vi "Shoot Joystick.vi"(6 "Auto Calculate Speed":bool, 8 "Trench Speed":bool, 9 "Init LIne Speed":bool, 10 "Target Zone Speed":bool, 11 "Raw Throttle":dbl) -> (3 "Shoot Teleop Command":T1)   [LabVIEW 2019]
uses:
  Shooter Mode Type Def.ctl
  Shooter Command Type Def.ctl
  Shooter Preset speeds Type Def.ctl
panel:
  # "AUTO CALCULATE DOES NOT DO\nANYTHING RIGHT NOW"
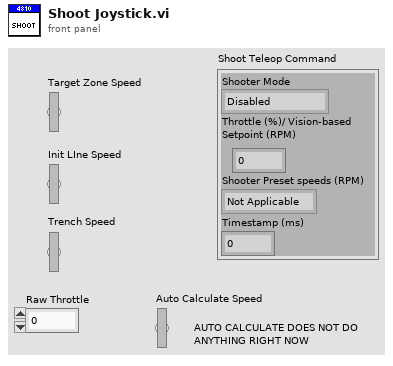
[diagram p1: front panel]
types:
  T1 = typedef "Shooter Command Type Def.ctl" = cluster{"Shooter Mode":T2, "Throttle (%)/ Vision-based\nSetpoint (RPM)":dbl, "Shooter Preset speeds (RPM)":T3, "Timestamp (ms)":dbl}
  T2 = typedef "Shooter Mode Type Def.ctl" = enum16{"Disabled", "Raw Throttle", "Preset Velocity Control", "Vision-based Velocity Control"}
  T3 = typedef "Shooter Preset speeds Type Def.ctl" = enum16{"Not Applicable", "Target Zone", "Initiation Line", "Close end of Trench Run", "Control Panel"}
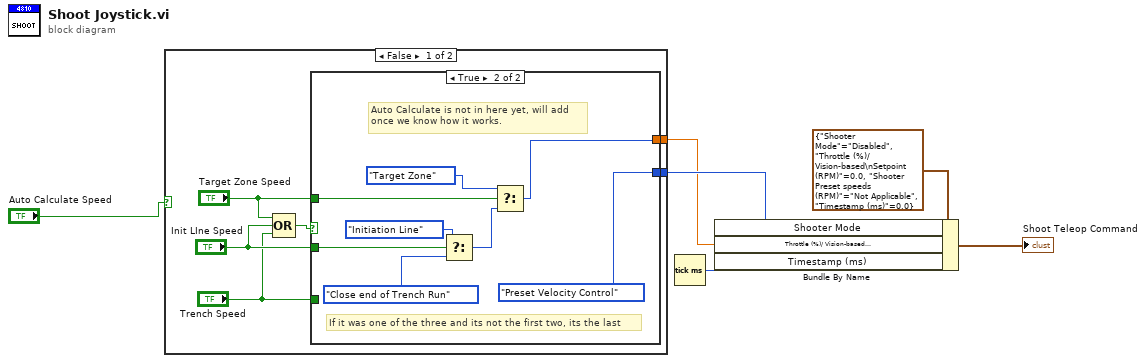
[diagram p0: block diagram]
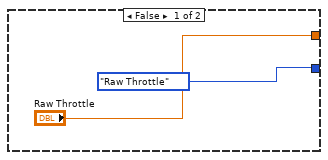
[diagram p2: hidden frame]
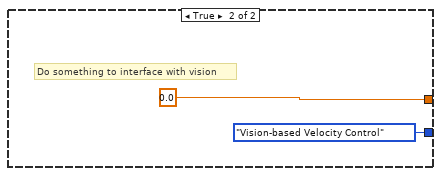
[diagram p3: hidden frame]
diagram:
  n1 = case shown="False" "Auto Calculate Speed" {
    tunnel: [w12 Shooter_Mode_Type_Def."Vision-based Velocity Control" ("Shooter Mode")] -> w3
    tunnel: [w7 0.0 ("Raw Throttle")] -> w2
    frame False {
      n2 = Compound Arithmetic op=OR("Target Zone Speed", "Init LIne Speed", "Trench Speed") -> (w11:bool)
      n3 = case shown="True" w11 {
        tunnel: "Trench Speed" -> [_ _]
        tunnel: "Init LIne Speed" -> [_ w22]
        tunnel: "Target Zone Speed" -> [_ w21]
        tunnel: [Shooter_Mode_Type_Def."Raw Throttle" ("Shooter Mode") Shooter_Mode_Type_Def."Preset Velocity Control" ("Shooter Mode")] -> w12
        tunnel: ["Raw Throttle" w19] -> w7
        frame False {
        }
        frame True {
          # "If it was one of the three and its not the first two, its the last"
          # "Auto Calculate is not in here yet, will add\nonce we know how it works."
          n4 = Select(t=Shooter_Preset_speeds_Type_Def."Initiation Line" ("Shooter Preset speeds (RPM)"), s=w22, f=Shooter_Preset_speeds_Type_Def."Close end of Trench Run" ("Shooter Preset speeds (RPM)")) -> (s? t:f=w20:T3)
          n5 = Select(t=Shooter_Preset_speeds_Type_Def."Target Zone" ("Shooter Preset speeds (RPM)"), s=w21, f=w20) -> (s? t:f=w19:T3)
        }
      }
    }
    frame True {
      # "Do something to interface with vision"
    }
  }
  n6 = Tick Count (ms)() -> (millisecond timer value=w4:u32)
  n7 = Bundle By Name(cluster=T1 {"Shooter Mode"=enum."Disabled", "Throttle (%)/ Vision-based\nSetpoint (RPM)"=0.0, "Shooter Preset speeds (RPM)"=enum."Not Applicable", "Timestamp (ms)"=0.0} ("Teleop Shooter Command"), "Shooter Mode"=w3, "Throttle (%)/ Vision-based\nSetpoint (RPM)"=w2, "Timestamp (ms)"=w4) -> (→"Shoot Teleop Command":T1)
